vi "Actuator_Characterisation.vi"() -> ()   [LabVIEW 2019]
uses:
  <vilib>/DAQmx/configure/timing.llb/DAQmx Timing (Sample Clock).vi
  <vilib>/DAQmx/create/channels.llb/DAQmx Create Channel (AI-Current-Basic).vi
  <vilib>/Utility/error.llb/DialogType.ctl
  <vilib>/DAQmx/read.llb/DAQmx Read (Analog DBL 1Chan 1Samp).vi
  <vilib>/measure/NI_MAPro.lvlib
  <vilib>/measure/maspectr.llb/FFT Power Spectrum and PSD for 1 Chan.vi
panel:
  out "data":dbl format="%0.2f"
  in  "stop":bool
  in  "physical channels":tag
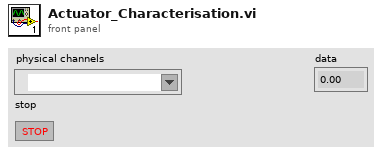
[diagram p1: front panel]
types:
  T1 = typedef "DialogType.ctl" = u16
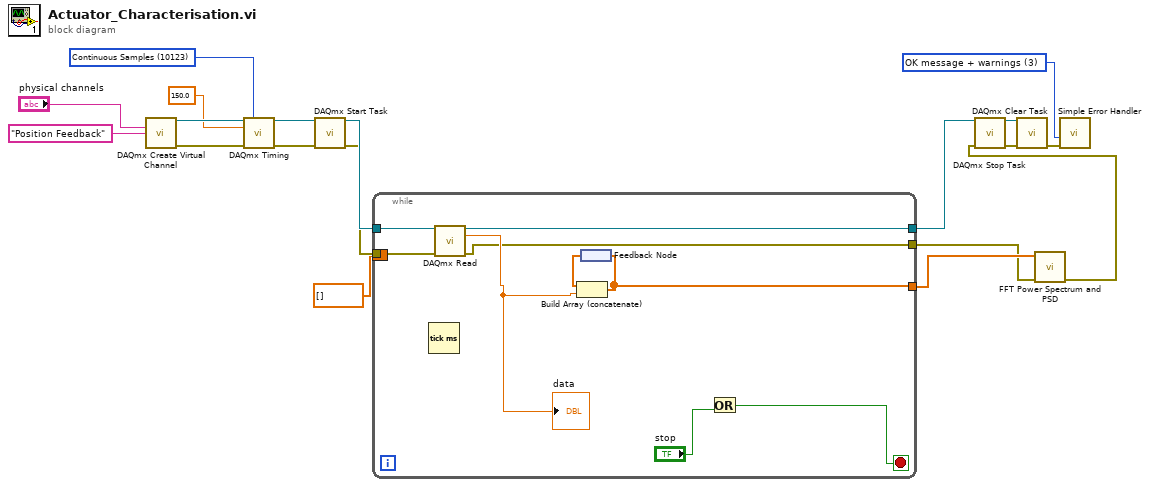
[diagram p0: block diagram]
diagram:
  w5 = T1 3 items=["no dialog", "OK message", "continue or stop message", "OK message + warnings", "continue/stop + warnings"] ("type of dialog (OK msg:1)")
  w11 = 10123 items=["Finite Samples"=10178, "Continuous Samples"=10123, "Hardware Timed Single Point"=12522] ("sample mode")
  n1 = call-poly <vilib>:"DAQmx Create Virtual Channel.vi"("physical channels"="physical channels", "name to assign"="Position Feedback") -> ("task out"=w19:refnum<k21>, "error out"=w18:errorcluster)  [unwired: 12 in]
  n2 = call-poly <vilib>:"DAQmx Timing.vi"("task/channels in"=w19, "sample mode"=w11, "rate"=150.0, "error in"=w18) -> ("task out"=w17:refnum<k21>, "error out"=w16:errorcluster)  [unwired: 10 in]
  n3 = call <vilib>:"DAQmx Start Task.vi"("task/channels in"=w17, "error in"=w16) -> ("task out"=w15:refnum<k21>, "error out"=w14:errorcluster)  [unwired: 12 in]
  n4 = while {
    tunnel: w15 -> [w26]
    tunnel: w14 -> [w28]
    tunnel: [w27] -> w9
    border: dbl[] [] -> [_]
    tunnel: [w21] -> w3
    tunnel: [w20] -> w2
    stop <- w24 stop-if-true
    n5 = Tick Count (ms)() -> ()  [unwired: 1 out]
    n6 = call-poly <vilib>:"DAQmx Read.vi"("task/channels in"=w26, "error in"=w28) -> ("task out"=w27:refnum<k21>, "data"=w23:dbl, "error out"=w20:errorcluster)  [unwired: 11 in]
    "data" <- w23
    n7 = feedback #1() -> (w22:dbl[])
    n8 = Build Array (concatenate)(w22, w23) -> (w21:dbl[])
    n9 = feedback-in #1(w21) -> ()
    n10 = Or(y="stop") -> (x .or. y?=w24:bool)  [unwired: 1 in]
  }
  n11 = call-poly <vilib>:"FFT Power Spectrum and PSD.vi"("error in (no error)"=w2, "time signal"=w3) -> ("error out"=w1:errorcluster)  [unwired: 6 in, 3 out]
  n12 = call <vilib>:"DAQmx Stop Task.vi"("task/channels in"=w9, "error in"=w1) -> ("task out"=w8:refnum<k21>, "error out"=w7:errorcluster)  [unwired: 12 in]
  n13 = call <vilib>:"DAQmx Clear Task.vi"("task in"=w8, "error in"=w7) -> ("error out"=w6:errorcluster)  [unwired: 13 in]
  n14 = call <vilib>:"Simple Error Handler.vi"("type of dialog (OK msg:1)"=w5, "error in (no error)"=w6) -> ()  [unwired: 3 in, 5 out]
